vi "Test Heart Rate calc.vi"() -> (2 "Heart Rate (bpm)":dbl format="%.1f")   [LabVIEW 2015]
uses:
  <vilib>/Analysis/2dsp.llb/Decimate (single shot, DBL).vi
  <vilib>/Analysis/NI_AALPro.lvlib
panel:
  in  "Path":path
  in  "Npts":u32=20000
  in  "Sampling Rate (Hz)":dbl=10000.0
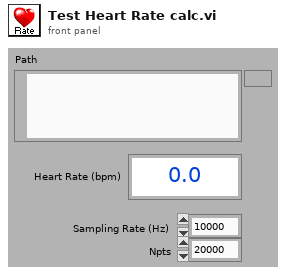
[diagram p1: front panel]
types:
  T1 = enum16{"open", "replace", "create", "open or create", "replace or create", "replace or create with confirmation"}
  T2 = enum16{"big-endian, network order", "native, host order", "little-endian"}
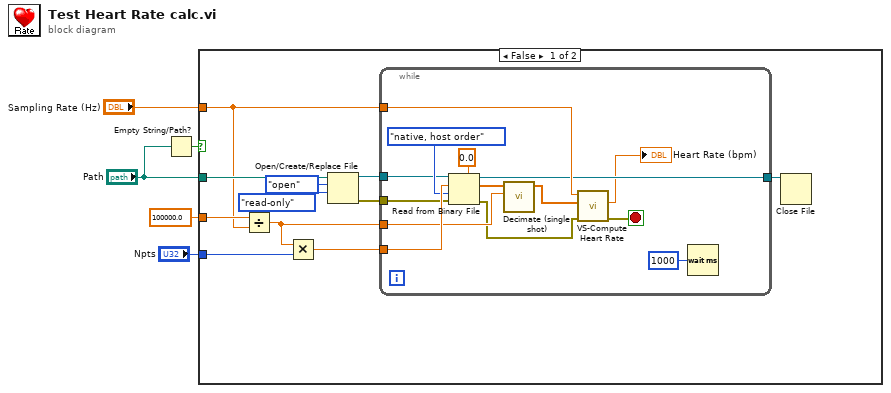
[diagram p0: block diagram]
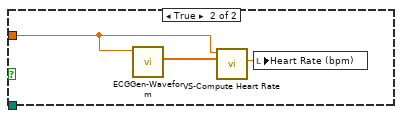
[diagram p2: hidden frame]
diagram:
  n1 = Empty String/Path?(string/path="Path") -> (empty?=w4:bool)
  n2 = case shown="False" w4 {
    tunnel: "Sampling Rate (Hz)" -> [w7 w32]
    tunnel: "Path" -> [w12 _]
    tunnel: 100000.0 -> [w16 _]
    tunnel: "Npts" -> [w15 _]
    frame False {
      n3 = Divide(x=w16, y=w7) -> (x/y=w13:dbl)
      n4 = Multiply(x=w13, y=w15) -> (x*y=w14:dbl)
      n5 = Open/Create/Replace File(file path (use dialog)=w12, operation (0:open)=T1."open", access (0:read/write)=enum16{"read/write", "read-only", "write-only"}."read-only") -> (refnum out=w11:refnum<file>, error out=w8:errorcluster)  [unwired: 3 in, 1 out]
      n6 = while {
        tunnel: w14 -> [w30]
        tunnel: w13 -> [w27]
        tunnel: w11 -> [w25]
        tunnel: w8 -> [w24]
        tunnel: w7 -> [w22]
        tunnel: [w19] -> w6
        stop <- w20 stop-if-true
        n7 = Read from Binary File(5:0.0, 8:w24, 9:T2."native, host order" ("byte order (0:big-endian, network order)"), 10:w30, 11:w25) -> (0:w21:errorcluster, 2:w28:dbl[], 3:w19:refnum<file>)  [unwired: 1 in, 1 out]
        n8 = call-poly <vilib>:"Decimate (single shot).vi"("decimating factor"=w27, "X"=w28) -> ("Decimated Array"=w23:dbl[])  [unwired: 8 in, 1 out]
        n9 = call "VS-Compute Heart Rate.vi"("error in (no error)"=w21, "ECG"=w23, "Sampling Rate (Hz)"=w22) -> ("error out"=w20:errorcluster, "Heart Rate (bpm)"=→"Heart Rate (bpm)":dbl)  [unwired: 7 in]
        n10 = Wait (ms)(milliseconds to wait=u32 1000) -> ()  [unwired: 1 out]
      }
      n11 = Close File(refnum=w6) -> ()  [unwired: 1 in, 2 out]
    }
    frame True {
      n12 = call "ECGGen-Waveform.vi"("Sampling Rate (Hz)"=w32) -> ("ECG Waveform"=w33:dbl[])  [unwired: 10 in]
      n13 = call "VS-Compute Heart Rate.vi"("ECG"=w33, "Sampling Rate (Hz)"=w32) -> ("Heart Rate (bpm)"=w31:dbl)  [unwired: 8 in, 1 out]
      n14 = local write "Heart Rate (bpm)"(w31) -> ()
    }
  }
